vi "Intan_ResumeSerialStream.vi"(11 "VISA resource name":refnum<visa-resource-name>="COM1") -> (0 "error out":errorcluster, 2 "Text response":string, 3 "VISA resource name out":refnum<visa-resource-name>)   [LabVIEW 2017]
panel:
  in  "bytes to read":u32=1000
  out "return count":u32
  in  "Teensy event char":string="u"
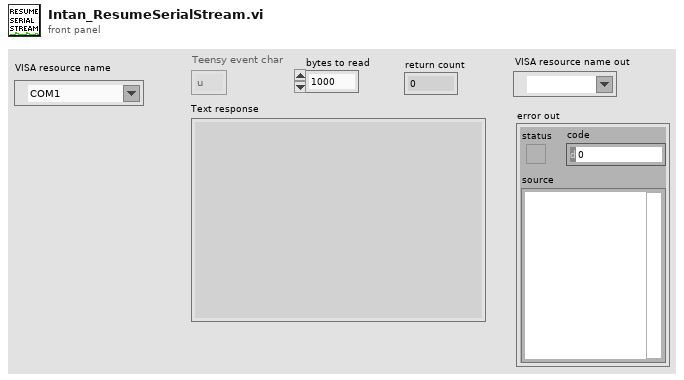
[diagram p1: front panel]
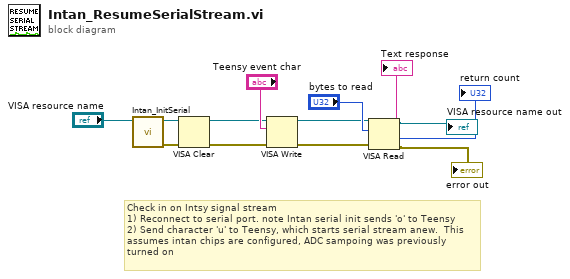
[diagram p0: block diagram]
diagram:
  # "Check in on Intsy signal stream\n1) Reconnect to serial port. note Intan serial init sends 'o' to Teensy\n2) Send character 'u' to Teensy, which starts serial stream anew.  This assumes intan chips are configured, ADC sampoing was previously turned on"
  n1 = call "Intan_InitSerial.vi"("VISA resource name"="VISA resource name") -> ("VISA resource name out"=w4:refnum<visa-resource-name>, "error out"=w3:errorcluster)  [unwired: 3 in, 1 out]
  n2 = VISA Clear(VISA resource name=w4, error in (no error)=w3) -> (VISA resource name out=w1:refnum<visa-resource-name>, error out=w2:errorcluster)
  n3 = VISA Write(VISA resource name=w1, write buffer="Teensy event char", error in (no error)=w2) -> (VISA resource name out=w8:refnum<visa-resource-name>, error out=w7:errorcluster)  [unwired: 1 out]
  n4 = VISA Read(VISA resource name=w8, byte count="bytes to read", error in (no error)=w7) -> (VISA resource name out=→"VISA resource name out":refnum<visa-resource-name>, read buffer=→"Text response":string, return count=→"return count":u32, error out=→"error out":errorcluster)
